vi "create_mission_waypoints.vi"(9 "Mission in":refnum<class "Mission.lvclass">) -> (1 "Mission out":refnum<class "Mission.lvclass">)   [LabVIEW 2011, in "Mission.lvclass"]
uses:
  Mission.lvclass
  Mission.lvclass/Mission.ctl
  2 Globals/2 Global.vi
  Waypoint/Waypoint.lvclass
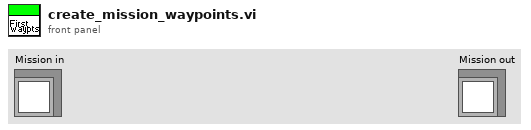
[diagram p1: front panel]
types:
  T1 = enum16{"Round Buoy", "Drive", "Pass Buoys", "Station Keeping"}
  T2 = typedef "UTM Location.ctl" = cluster{"UTM Zone":dbl, "Hemisphere":enum16{"North", "South"}, "East":dbl, "North":dbl}
  T3 = typedef "Waypoints List.ctl" = refnum<class "Waypoint.lvclass">[]
  T4 = typedef "UTM Circle.ctl" = cluster{"UTM Zone":dbl, "Hemisphere":enum16{"North", "South"}, "East":dbl, "North":dbl, "Radius":dbl}
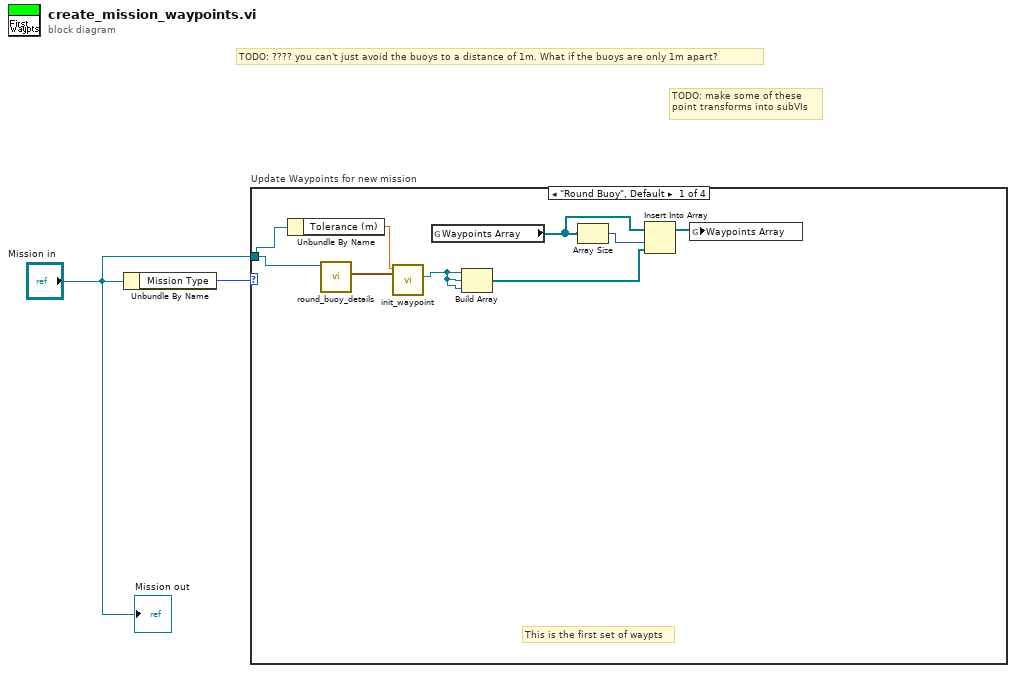
[diagram p0: block diagram]
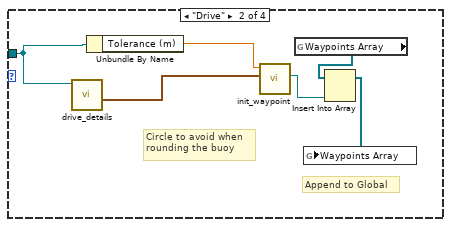
[diagram p2: hidden frame]
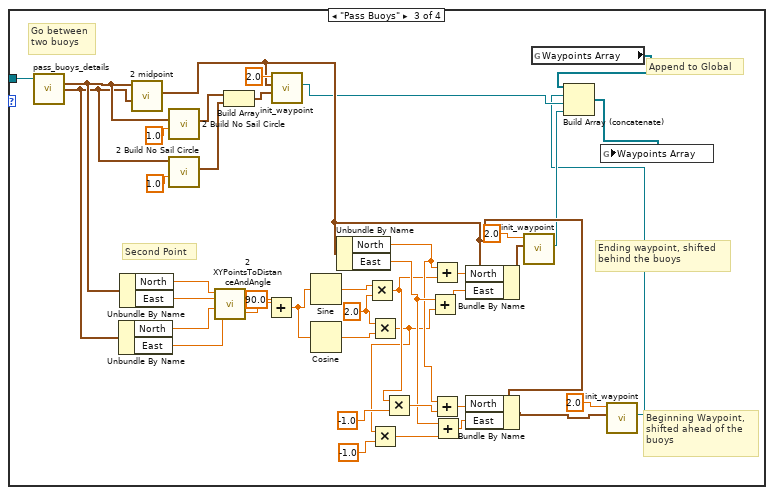
[diagram p3: hidden frame]
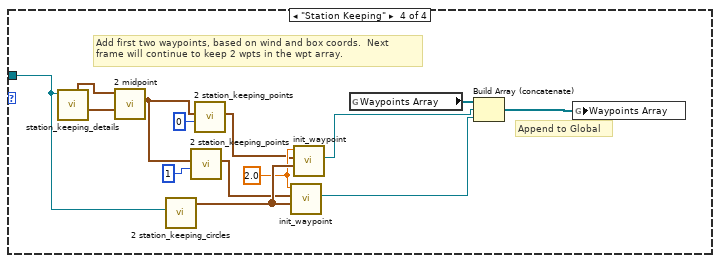
[diagram p4: hidden frame]
diagram:
  # "TODO: make some of these\npoint transforms into subVIs"
  # "TODO: ???? you can't just avoid the buoys to a distance of 1m. What if the buoys are only 1m apart?"
  n1 = Unbundle By Name("Mission in") -> ("Mission Type"=w2:T1)
  n2 = case "Update Waypoints for new mission" shown="\"Round Buoy\", Default" w2 {
    tunnel: "Mission in" -> [w3 w12 w53 w66]
    frame "Round Buoy", Default {
      # "This is the first set of waypts"
      n3 = Unbundle By Name(w3) -> ("Tolerance (m)"=w4:dbl)
      n4 = call-dynamic "round_buoy_details.vi"("Mission in"=w3) -> ("Buoy to Round"=w10:T2)  [unwired: 7 in, 3 out]
      n5 = call "init_waypoint.vi"("Coords"=w10, "Tolerance (m)"=w4) -> ("Waypoint Out"=w9:refnum<class "Waypoint.lvclass">)  [unwired: 9 in]
      n6 = global read "2 Global.vi" "Waypoints Array"() -> (w7:T3)
      n7 = Build Array(w9, w9, w9) -> (w6:refnum<class "Waypoint.lvclass">[])
      n8 = Array Size(array=w7) -> (size(s)=w8:i32)
      n9 = Insert Into Array(array=w7, index=w8, new element=w6) -> (w5:T3)
      n10 = global write "2 Global.vi" "Waypoints Array"(w5) -> ()
    }
    frame "Drive" {
      # "Append to Global"
      # "Circle to avoid when\nrounding the buoy"
      n11 = call-dynamic "drive_details.vi"("Mission in"=w12) -> ("Drive Location"=w14:T2)  [unwired: 8 in, 2 out]
      n12 = Unbundle By Name(w12) -> ("Tolerance (m)"=w11:dbl)
      n13 = call "init_waypoint.vi"("Coords"=w14, "Tolerance (m)"=w11) -> ("Waypoint Out"=w13:refnum<class "Waypoint.lvclass">)  [unwired: 9 in]
      n14 = global read "2 Global.vi" "Waypoints Array"() -> (w15:T3)
      n15 = Insert Into Array(array=w15, new element=w13) -> (w16:T3)  [unwired: 1 in]
      n16 = global write "2 Global.vi" "Waypoints Array"(w16) -> ()
    }
    frame "Pass Buoys" {
      w33 = 2.0 ("Tolerance (meters?)")
      # "Ending waypoint, shifted\nbehind the buoys"
      # "Beginning Waypoint,\nshifted ahead of the\nbuoys"
      # "Second Point"
      # "Go between\ntwo buoys"
      # "Append to Global"
      n17 = call-dynamic "pass_buoys_details.vi"("Mission in"=w53) -> ("Buoy Pass Port"=w48:T2, "Buoy Pass Starboard"=w47:T2)  [unwired: 11 in, 2 out]
      n18 = Unbundle By Name(w47) -> ("North"=w44:dbl, "East"=w43:dbl)
      n19 = Unbundle By Name(w48) -> ("North"=w46:dbl, "East"=w45:dbl)
      n20 = call "2 midpoint.vi"("UTM 2"=w47, "UTM 1"=w48) -> ("Midpoint"=w22:T2)  [unwired: 8 in, 1 out]
      n21 = call "2 Build No Sail Circle.vi"("Radius"=1.0, "UTM Location"=w48) -> ("UTM Circle"=w56:T4)  [unwired: 9 in]
      n22 = call "2 Build No Sail Circle.vi"("Radius"=1.0, "UTM Location"=w47) -> ("UTM Circle"=w52:T4)  [unwired: 9 in]
      n23 = call "2 XYPointsToDistanceAndAngle.vi"("East 2"=w43, "North 2"=w44, "East 1"=w45, "North 1"=w46) -> ("Angle Diff"=w42:dbl)  [unwired: 1 out]
      n24 = Build Array(w56, w52) -> (w57:T4[])
      n25 = Add(x=w42, y=90.0 ("Radius")) -> (x+y=w40:dbl)
      n26 = call "init_waypoint.vi"("No Sail Circles"=w57, "Coords"=w22, "Tolerance (m)"=2.0 ("Tolerance (meters?)")) -> ("Waypoint Out"=w18:refnum<class "Waypoint.lvclass">)  [unwired: 8 in]
      n27 = Sine(x=w40) -> (sin(x)=w35:dbl)
      n28 = Cosine(x=w40) -> (cos(x)=w34:dbl)
      n29 = Unbundle By Name(w22) -> ("North"=w27:dbl, "East"=w28:dbl)
      n30 = Multiply(x=w35, y=w33) -> (x*y=w26:dbl)
      n31 = Multiply(x=w33, y=w34) -> (x*y=w25:dbl)
      n32 = Multiply(x=w25, y=-1.0 ("Tolerance (meters?)")) -> (x*y=w30:dbl)
      n33 = Multiply(x=w26, y=-1.0 ("Tolerance (meters?)")) -> (x*y=w29:dbl)
      n34 = Add(x=w28, y=w25) -> (x+y=w39:dbl)
      n35 = Add(x=w27, y=w26) -> (x+y=w38:dbl)
      n36 = Add(x=w27, y=w29) -> (x+y=w24:dbl)
      n37 = Add(x=w28, y=w30) -> (x+y=w23:dbl)
      n38 = Bundle By Name(cluster=w22, "North"=w38, "East"=w39) -> (w37:T2)
      n39 = Bundle By Name(cluster=w22, "North"=w24, "East"=w23) -> (w20:T2)
      n40 = call "init_waypoint.vi"("Coords"=w37, "Tolerance (m)"=2.0 ("Tolerance (meters?)")) -> ("Waypoint Out"=w19:refnum<class "Waypoint.lvclass">)  [unwired: 9 in]
      n41 = global read "2 Global.vi" "Waypoints Array"() -> (w50:T3)
      n42 = call "init_waypoint.vi"("Coords"=w20, "Tolerance (m)"=2.0 ("Tolerance (meters?)")) -> ("Waypoint Out"=w17:refnum<class "Waypoint.lvclass">)  [unwired: 9 in]
      n43 = Build Array (concatenate)(w50, w17, w18, w19) -> (w49:T3)
      n44 = global write "2 Global.vi" "Waypoints Array"(w49) -> ()
    }
    frame "Station Keeping" {
      w64 = 2.0 ("Tolerance (meters?)")
      # "Append to Global"
      # "Add first two waypoints, based on wind and box coords.  Next\nframe will continue to keep 2 wpts in the wpt array."
      n45 = call-dynamic "station_keeping_details.vi"("Mission in"=w66) -> ("Buoy SE"=w70:T2, "Buoy NW"=w71:T2)  [unwired: 4 in, 5 out]
      n46 = call "2 midpoint.vi"("UTM 2"=w70, "UTM 1"=w71) -> ("Midpoint"=w61:T2)  [unwired: 8 in, 1 out]
      n47 = call "2 station_keeping_circles.vi"("Mission in"=w66) -> ("No Sail Circles"=w65:T4[])  [unwired: 10 in]
      n48 = call "2 station_keeping_points.vi"("Which Point?"=1, "Midpoint"=w61) -> ("Waypoint"=w63:T2)  [unwired: 9 in]
      n49 = call "2 station_keeping_points.vi"("Which Point?"=0, "Midpoint"=w61) -> ("Waypoint"=w62:T2)  [unwired: 9 in]
      n50 = call "init_waypoint.vi"("No Sail Circles"=w65, "Coords"=w63, "Tolerance (m)"=w64) -> ("Waypoint Out"=w67:refnum<class "Waypoint.lvclass">)  [unwired: 8 in]
      n51 = call "init_waypoint.vi"("No Sail Circles"=w65, "Coords"=w62, "Tolerance (m)"=w64) -> ("Waypoint Out"=w68:refnum<class "Waypoint.lvclass">)  [unwired: 8 in]
      n52 = global read "2 Global.vi" "Waypoints Array"() -> (w69:T3)
      n53 = Build Array (concatenate)(w69, w68, w67) -> (w58:T3)
      n54 = global write "2 Global.vi" "Waypoints Array"(w58) -> ()
    }
  }
  "Mission out" <- "Mission in"
